vi "racunanje ddQ.vi"(6 "T":T1, 9 "dQ":T1, 10 "g":dbl, 11 "Q":T1) -> (3 "ddQ":T1)   [LabVIEW 2014]
uses:
  <vilib>/Analysis/Matrix/Datatypes/RealMatrix.ctl
  <vilib>/Analysis/baseanly.llb/Real A x B.vi
  <vilib>/Analysis/Matrix/Numeric/Add/Add.vi
  <vilib>/Analysis/Matrix/Numeric/Add/Add - RM,RM.vi
  <vilib>/Analysis/Matrix/Numeric/Multiply/Multiply - R,RM.vi
  <vilib>/Analysis/Matrix/NI_Matrix.lvlib
  <vilib>/Analysis/NI_AALBase.lvlib
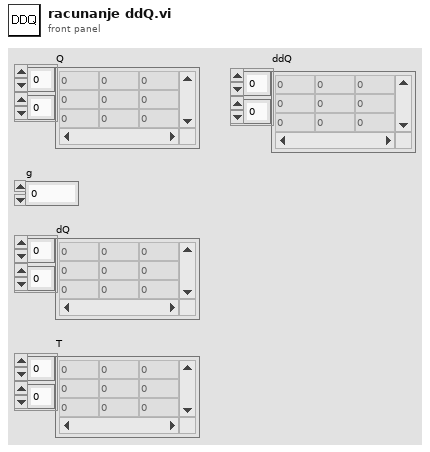
[diagram p1: front panel]
types:
  T1 = typedef "NI_Matrix.lvlib/RealMatrix.ctl" = dbl[][]
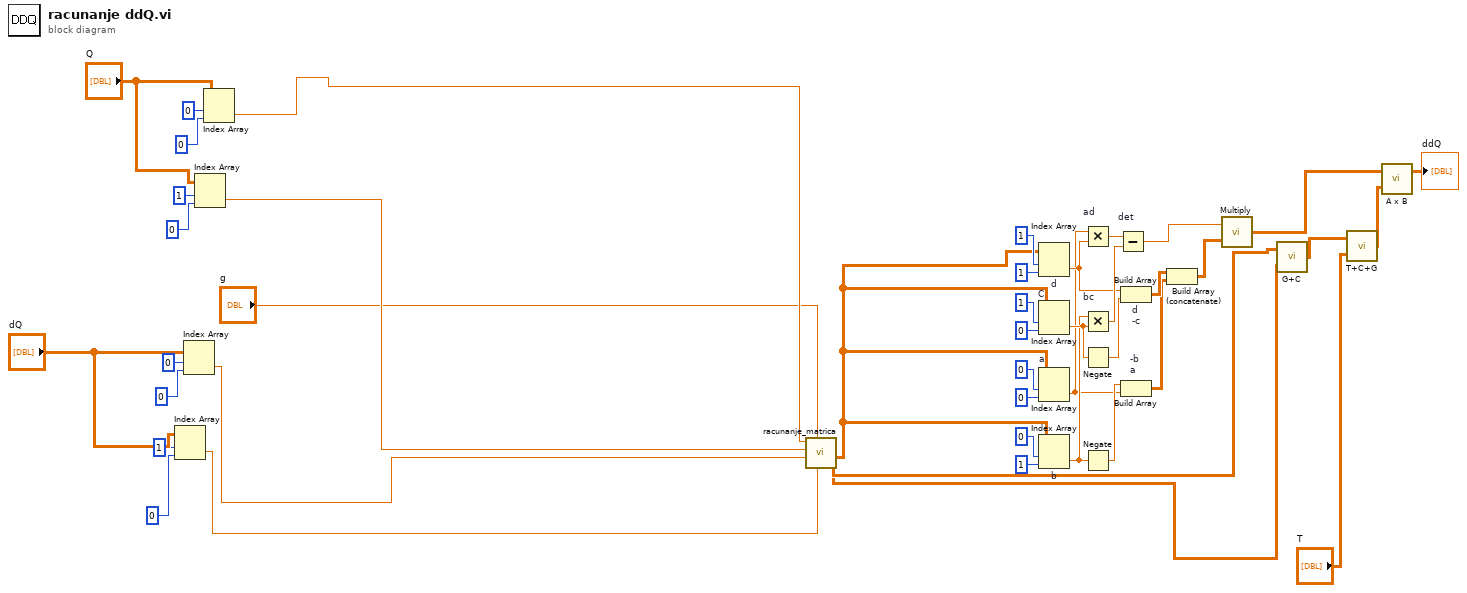
[diagram p0: block diagram]
diagram:
  n1 = Index Array(array="dQ", index (row)=1, index (col)=0 ("index (row)")) -> (element=w42:dbl)
  n2 = Index Array(array="dQ", index (row)=0, index (col)=0 ("index (row)")) -> (element=w40:dbl)
  n3 = Index Array(array="Q", index (row)=1, index (col)=0 ("index (row)")) -> (element=w35:dbl)
  n4 = Index Array(array="Q", index (row)=0, index (col)=0 ("index (row)")) -> (element=w32:dbl)
  n5 = call "racunanje_matrica.vi"("dq2"=w42, "g"="g", "dq1"=w40, "q2"=w35, "q1"=w32) -> ("M"=w2:T1, "G"=w24:T1, "C"=w28:T1)  [unwired: 4 in]
  n6 = Index Array "d"(array=w2, index (row)=1, index (col)=1) -> (element=w10:dbl)
  n7 = Index Array "C"(array=w2, index (row)=1, index (col)=0) -> (element=w8:dbl)
  n8 = Index Array "a"(array=w2, index (row)=0, index (col)=0) -> (element=w5:dbl)
  n9 = Index Array "b"(array=w2, index (row)=0, index (col)=1) -> (element=w6:dbl)
  n10 = Multiply "ad"(x=w5, y=w10) -> (x*y=w14:dbl)
  n11 = Multiply "bc"(x=w6, y=w8) -> (x*y=w13:dbl)
  n12 = Negate(x=w8) -> (-x=w9:dbl)
  n13 = Negate(x=w6) -> (-x=w7:dbl)
  n14 = Subtract "det"(x=w14, y=w13) -> (x-y=w3:dbl)
  n15 = Build Array "d\n-c"(w10, w9) -> (w12:T1)
  n16 = Build Array "-b\na"(w7, w5) -> (w11:T1)
  n17 = Build Array (concatenate)(w12, w11) -> (w4:T1)
  n18 = call-poly <vilib>:"Multiply.vi"("Real Matrix A"=w4, "Real Scalar c"=w3) -> ("c * A"=w1:T1)
  n19 = call-poly "G+C"("Real Matrix B"=w24, "Real Matrix A"=w28) -> ("A + B"=w25:T1)
  n20 = call-poly "T+C+G"("Real Matrix B"="T", "Real Matrix A"=w25) -> ("A + B"=w27:T1)
  n21 = call-poly <vilib>:"A x B.vi"("B"=w27, "A"=w1) -> ("A x B"=→"ddQ":T1)  [unwired: 1 out]
